vi "Get Port HW Entry by id.vi"(9 "port":u32, 10 "board":u32, 11 "hw_data in":T2) -> (1 "port hw entry out":T1, 2 "key not found?":bool, 3 "hw_data out":T2)   [LabVIEW 2020, in "AIM664LV.lvlib"]
uses:
  AIM664LV.lvlib
  _controls/hwEntry_data.ctl
  _controls/hwEntryBoardHandleMap.ctl
  _controls/hwEntryBoardResource.ctl
  _controls/hwEntryPortResource.ctl
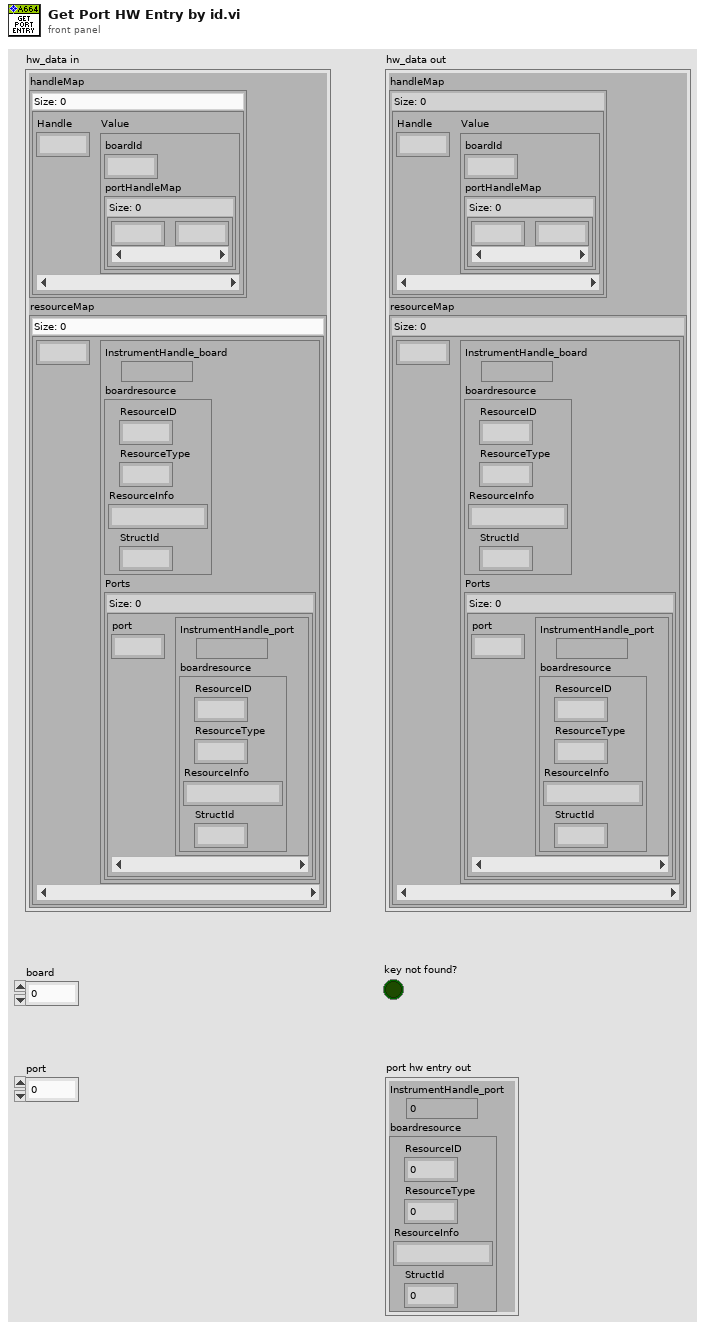
[diagram p1: front panel]
types:
  T1 = typedef "AIM664LV.lvlib/hwEntryPortResource.ctl" = cluster{"InstrumentHandle_port":u32, "boardresource":cluster{"ResourceID":u32, "ResourceType":u32, "ResourceInfo":string, "StructId":u32}}
  T2 = typedef "AIM664LV.lvlib/hwEntry_data.ctl" = cluster{"handleMap":map{u32, T3}, "resourceMap":map{u32, T4}}
  T3 = typedef "AIM664LV.lvlib/hwEntryBoardHandleMap.ctl" = cluster{"boardId":u32, "portHandleMap":map{u32, u32}}
  T4 = typedef "AIM664LV.lvlib/hwEntryBoardResource.ctl" = cluster{"InstrumentHandle_board":u32, "boardresource":cluster{"ResourceID":u32, "ResourceType":u32, "ResourceInfo":string, "StructId":u32}, "Ports":map{u32, T1}}
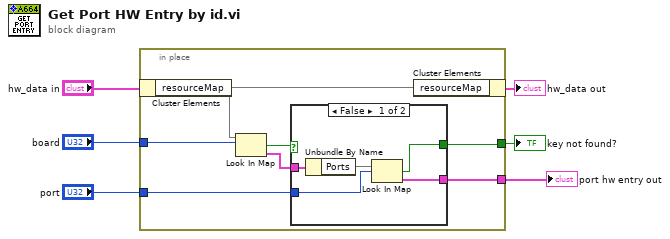
[diagram p0: block diagram]
diagram:
  n1 = in-place {
    in-place-border: "board" -> [w12]
    in-place-border: [w9] -> w3
    in-place-border: "port" -> [w8]
    in-place-border: [w7] -> w1
    n2 = in-place-cluster #1("hw_data in") -> ("resourceMap"=w13:map{u32, T4})
    n3 = Look In Map(map=w13, key=w12) -> (key not found?=w10:bool, value=w11:T4)  [unwired: 1 in]
    n4 = case shown="False" w10 {
      selector: w10 -> [_ w19]
      tunnel: w11 -> [w18 _]
      tunnel: [w14 w19] -> w9
      tunnel: w8 -> [w16 _]
      tunnel: [w15 _] -> w7
      frame False {
        n5 = Unbundle By Name(w18) -> ("Ports"=w17:map{u32, T1})
        n6 = Look In Map(map=w17, key=w16) -> (key not found?=w14:bool, value=w15:T1)  [unwired: 1 in]
      }
      frame True {
      }
    }
    n7 = in-place-cluster #1("resourceMap"=w13) -> (→"hw_data out":T2)
  }
  "key not found?" <- w3
  "port hw entry out" <- w1
